vi "VI-File-Explorer_Folder.vi"() -> ()   [LabVIEW 2021, in "vi_lib.lvlib"]
uses:
  vi_lib.lvlib
  clLabview/clLabview.lvclass
  clFile/clFile.lvclass
  <userlib>/John_Lib/TopPath/TopPath.lvlib
panel:
  out "lowercase file extension":string
  out "size(s)":i32
  out "Path":path
  out "Numeric":i32
  out "concatenated string":string
  in  "new VI-Lib Password":string
  in  "Update LV-Lib Password":bool
  out "File is protected?":bool=TRUE
  out "LV-Lib password (Hex)":string
  out "Icon":picture
  out "busy (*)":bool
  out "Salt (Hex)":string
  out "MD5-Hash 2 (Hex)":string
  out "MD5-Hash 1 (Hex)":string
  out "saving done":bool
  in  "save":bool
  in  "Open":bool
  in  "stop":bool
  out "flags":i32 step=1
  out "stage":u8(ring) items=["development", "alpha", "beta", "release"]
  out "build":u8 step=1
  out "bugfix":u8 step=1
  out "minor":u8 max=99 step=1
  out "major":u8=3 min=1 max=99 step=1
  out "version info":string
  out "version text":string
  in  "save to":path=path "D:/labview/file_in_(free).vi"
  in  "new File Password":string
  in  "open from":path=path "D:/labview/file.vi"
  out "MD5 password (Hex)":string
  # "MD5 password (Hex)\nMD5-Hash 1 (Hex)\nMD5-Hash 2 (Hex) for LV-Version >= 8\nLV-Lib password (Hex)"
  # "File password [BDPW]"
  # "for LV-Version >= 8"
  # "for LV-Version >= 12"
  # "(*) This is a \"brute force\" version to calc the password Salt, \n      so it might take up to 30sec."
  # "File propertys [LVSR]"
  # "File version [vers]"
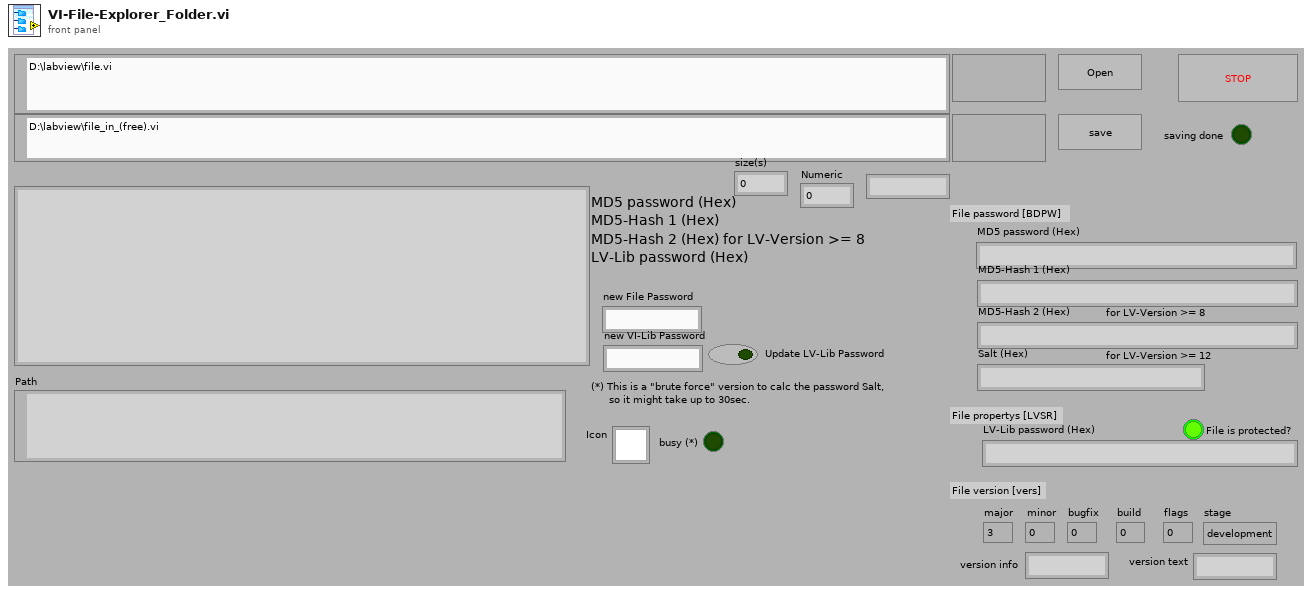
[diagram p1: front panel]
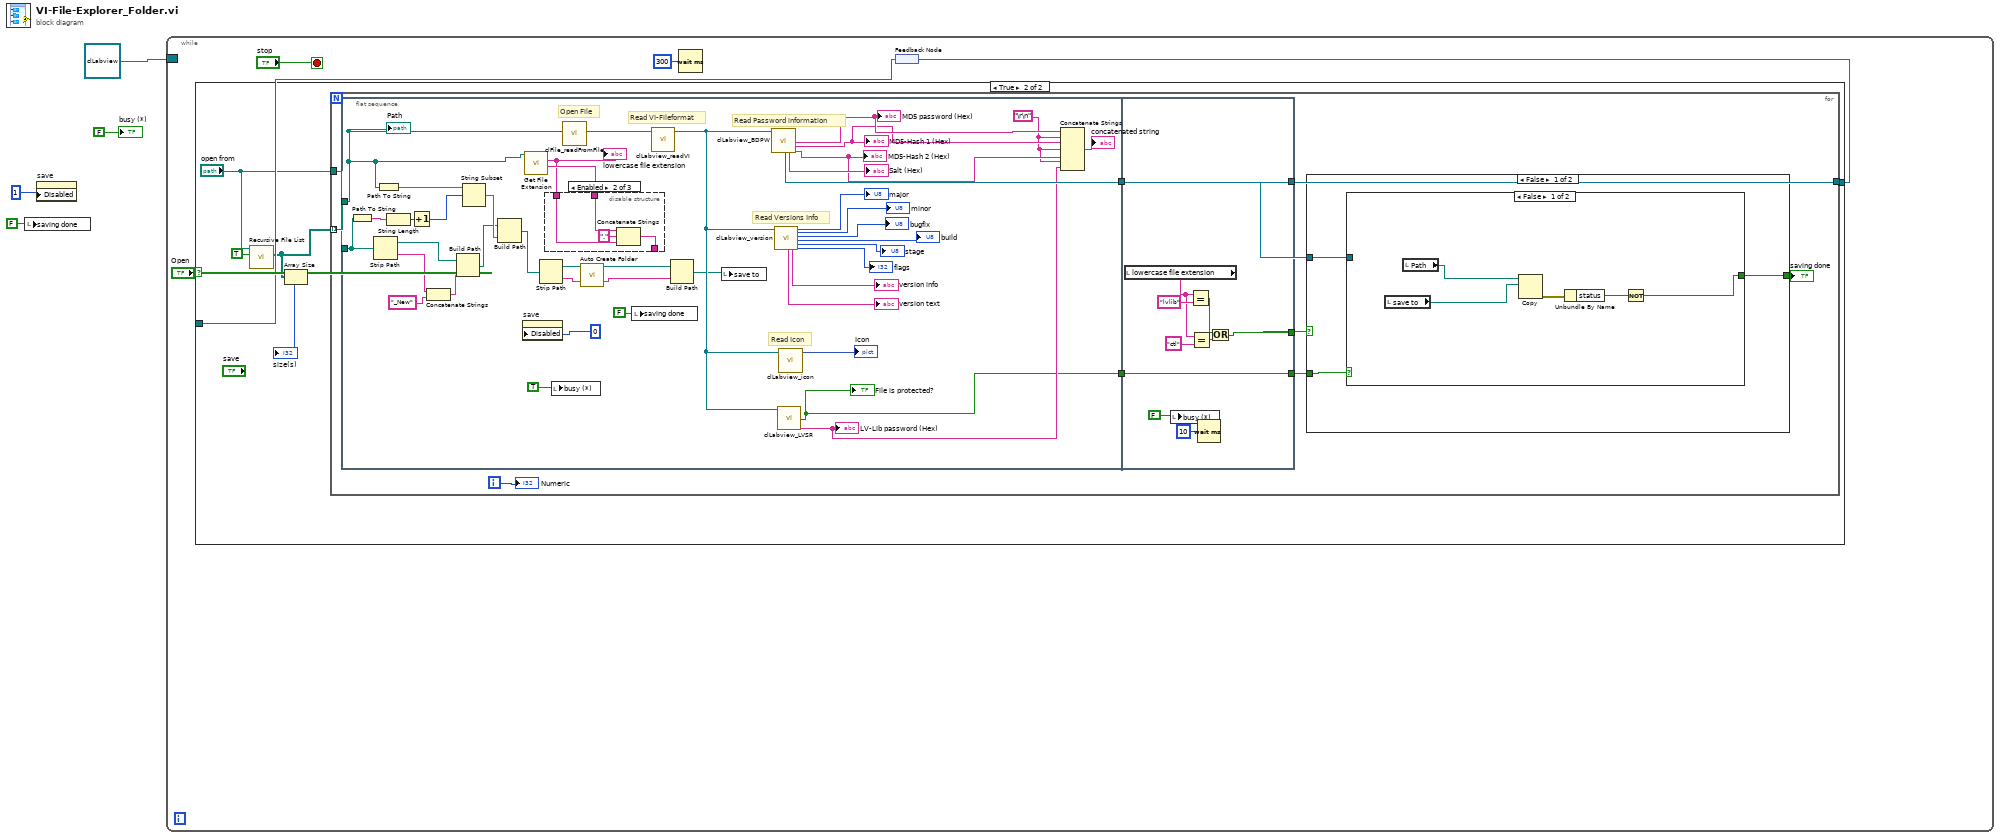
[diagram p0: block diagram]
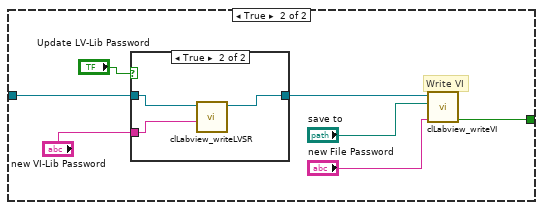
[diagram p3: hidden frame]
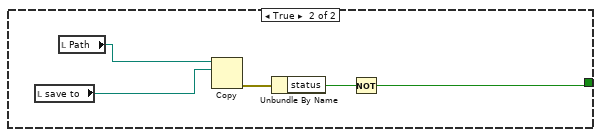
[diagram p5: hidden frame]
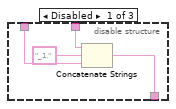
[diagram p6: hidden frame]
diagram:
  n1 = local write "saving done"(FALSE ("saving done")) -> ()
  n2 = property on="save" class="Bool"("Disabled"=u8 1) -> ()  [unwired: 2 in, 2 out]
  n3 = while {
    border: refnum<class "clLabview.lvclass"> refnum ("vi_lib.lvlib:clLabview.lvclass 2") -> [_]
    stop <- "stop" stop-if-true
    n4 = Wait (ms)(milliseconds to wait=u32 300) -> ()  [unwired: 1 out]
    n5 = feedback #1() -> (w5:refnum<class "clLabview.lvclass">)
    n6 = case shown="True" "Open" {
      tunnel: [w10 w15] -> w7
      tunnel: w5 -> [w10 _]
      frame False {
      }
      frame True {
        n7 = call <vilib>:"Recursive File List.vi"("Treat LLBs as Folders?"=TRUE, "Folder Path"="open from") -> ("All Files in Dir"=w12:path[])  [unwired: 5 in, 4 out]
        n8 = Array Size(array=w12) -> (size(s)=→"size(s)":i32)
        n9 = for {
          tunnel: [w23] -> w15
          tunnel: w12 -> [w22] mode=indexing
          tunnel: "open from" -> [w20]
          i -> [w21]
          n10 = flat-sequence {
            tunnel: [w79] -> w24
            tunnel: w22 -> [w60]
            tunnel: w20 -> [w59]
            tunnel: [w49] -> w17
            tunnel: [w108] -> w23
            tunnel: w24 -> [w108]
            tunnel: [w100] -> w19
            tunnel: w17 -> [w99]
            tunnel: [w99] -> w16
            frame #0 {
              w68 = "\r\n"
              # "Read Icon"
              # "Read Versions Info"
              # "Read Password information"
              # "Read VI-Fileformat"
              # "Open File"
              n11 = Path To String(path=w59) -> (string=w57:string)
              n12 = Strip Path(path=w59) -> (stripped path=w63:path, name=w62:string)
              n13 = Path To String(path=w60) -> (string=w58:string)
              n14 = String Length(string=w57) -> (length=w51:i32)
              n15 = Increment(x=w51) -> (x+1=w50:i32)
              n16 = Concatenate Strings(w62, "_New" ("string")) -> (w65:string)
              n17 = Build Path(base path=w63, name or relative path=w65) -> (appended path=w54:path)
              n18 = String Subset(string=w58, offset (0)=w50) -> (substring=w56:string)  [unwired: 1 in]
              n19 = Build Path(base path=w54, name or relative path=w56) -> (appended path=w55:path)
              n20 = property on="save" class="Bool"("Disabled"=u8 0) -> ()  [unwired: 2 in, 2 out]
              n21 = call <vilib>:"Get File Extension.vi"("file"=w60) -> ("filename without extension"=w74:string, "lowercase file extension"=w73:string)  [unwired: 6 in, 3 out]
              "lowercase file extension" <- w73
              n22 = Strip Path(path=w55) -> (stripped path=w53:path, name=w52:string)
              n23 = disable-structure shown="Enabled" {
                disable-tunnel: w74 -> [w94 w98 _]
                disable-tunnel: w73 -> [w92 w97 _]
                disable-tunnel: [w91 w96 _] -> _
                frame Disabled {
                  n24 = Concatenate Strings(w94, "_1." ("string"), w92) -> (w91:string)
                }
                frame Enabled {
                  n25 = Concatenate Strings(w98, "." ("string"), w97) -> (w96:string)
                }
                frame Disabled {
                }
              }
              n26 = local write "busy (*)"(TRUE ("busy")) -> ()
              n27 = call "clFile_readFromFile.vi"("file (use dialog)"=w60) -> ("clFileReader.lvclass"=w90:refnum<class "clFileReader.lvclass">)  [unwired: 1 in, 9 out]
              n28 = call <userlib>:"Auto Create Folder.vi"("Folder path"=w53) -> ("Folder path"=w61:path)  [unwired: 9 in, 1 out]
              n29 = local write "saving done"(FALSE ("saving done")) -> ()
              n30 = call "clLabview_readVI.vi"("vi_lib.lvlib:clFileReader.lvclass"=w90) -> ("vi_lib.lvlib:clLabview.lvclass 2"=w76:refnum<class "clLabview.lvclass">)  [unwired: 10 out]
              n31 = Build Path(base path=w61, name or relative path=w52) -> (appended path=w75:path)
              n32 = local write "save to"(w75) -> ()
              n33 = call "clLabview_BDPW.vi"("vi_lib.lvlib:clLabview.lvclass"=w76) -> ("vi_lib.lvlib:clLabview.lvclass [Out]"=w79:refnum<class "clLabview.lvclass">, "Salt (Hex)"=→"Salt (Hex)":string, "MD5 password (Hex)"=w72:string, "MD5-Hash 1  (Hex)"=w71:string, "MD5-Hash 2  (Hex)"=w70:string)  [unwired: 14 out]
              "MD5 password (Hex)" <- w72
              "MD5-Hash 2 (Hex)" <- w70
              "MD5-Hash 1 (Hex)" <- w71
              n34 = call "clLabview_version.vi"("vi_lib.lvlib:clLabview.lvclass"=w76) -> ("version_text"=→"version text":string, "version_info"=→"version info":string, "major"=→"major":u8, "minor"=→"minor":u8, "bugfix"=→"bugfix":u8, "build"=→"build":u8, "stage"=→"stage":u8, "flags"=→"flags":i32)  [unwired: 11 out]
              n35 = call "clLabview_LVSR.vi"("vi_lib.lvlib:clLabview.lvclass"=w76) -> ("File is protected?"=w49:bool, "MD5 lib Password (Hex)"=w67:string)  [unwired: 17 out]
              "LV-Lib password (Hex)" <- w67
              "File is protected?" <- w49
              n36 = call "clLabview_icon.vi"("vi_lib.lvlib:clLabview.lvclass"=w76) -> ("Icon"=→"Icon":picture)  [unwired: 10 out]
              n37 = Concatenate Strings(w72, w68, w71, w68, w70, w68, w67) -> (→"concatenated string":string)
              "Path" <- w60
            }
            frame #1 {
              n38 = local read "lowercase file extension"() -> (w102:string)
              n39 = local write "busy (*)"(FALSE ("busy")) -> ()
              n40 = Equal?(x=w102, y="lvlib") -> (x = y?=w104:bool)
              n41 = Equal?(x=w102, y="ctl") -> (x = y?=w101:bool)
              n42 = Wait (ms)(milliseconds to wait=u32 10) -> ()  [unwired: 1 out]
              n43 = Or(x=w104, y=w101) -> (x .or. y?=w100:bool)
            }
          }
          n44 = case shown="False" w19 {
            tunnel: w23 -> [w27 _]
            tunnel: [w26 w44] -> w18
            tunnel: w16 -> [w25 _]
            frame False {
              n45 = case shown="False" w25 {
                tunnel: w27 -> [_ w39]
                tunnel: [w28 w38] -> w26
                frame False {
                  n46 = local read "save to"() -> (w31:path)
                  n47 = local read "Path"() -> (w32:path)
                  n48 = Copy(10:w31, 11:w32) -> (0:w30:errorcluster)  [unwired: 3 in, 2 out]
                  n49 = Unbundle By Name(w30) -> ("status"=w29:bool)
                  n50 = Not(x=w29) -> (.not. x?=w28:bool)
                }
                frame True {
                  # "Write VI"
                  n51 = case shown="True" "Update LV-Lib Password" {
                    tunnel: w39 -> [w40 w43]
                    tunnel: [w40 w42] -> w35
                    tunnel: "new VI-Lib Password" -> [_ w41]
                    frame False {
                    }
                    frame True {
                      n52 = call "clLabview_writeLVSR.vi"("vi_lib.lvlib:clLabview.lvclass"=w43, "new lib Password"=w41) -> ("vi_lib.lvlib:clLabview.lvclass [Out]"=w42:refnum<class "clLabview.lvclass">)  [unwired: 8 out]
                    }
                  }
                  n53 = call "clLabview_writeVI.vi"("vi_lib.lvlib:clLabview.lvclass"=w35, "filename (use dialog)"="save to", "new Password"="new File Password") -> ("no Error"=w38:bool)  [unwired: 7 out]
                }
              }
            }
            frame True {
              n54 = local read "save to"() -> (w47:path)
              n55 = local read "Path"() -> (w48:path)
              n56 = Copy(10:w47, 11:w48) -> (0:w46:errorcluster)  [unwired: 3 in, 2 out]
              n57 = Unbundle By Name(w46) -> ("status"=w45:bool)
              n58 = Not(x=w45) -> (.not. x?=w44:bool)
            }
          }
          "saving done" <- w18
          "Numeric" <- w21
        }
      }
    }
    n59 = feedback-in #1(w7) -> ()
  }
  "busy (*)" <- FALSE ("busy")
